vi "OAT Get Orbit Precession Direction.vi"(8 "error in (no error)":errorcluster, 9 "shaft rotating direction":u16, 10 "max data value":dbl format="%.2f", 11 "XY plot data in":cluster{dbl[], dbl[]}[](array[cluster]) {"?" format="%.2f"; "?" format="%.2f"}) -> (0 "error out":errorcluster, 3 "XY plot data out":cluster{dbl[], dbl[]}[](array[cluster]) {"?" format="%.2f"; "?" format="%.2f"})   [LabVIEW 2017]
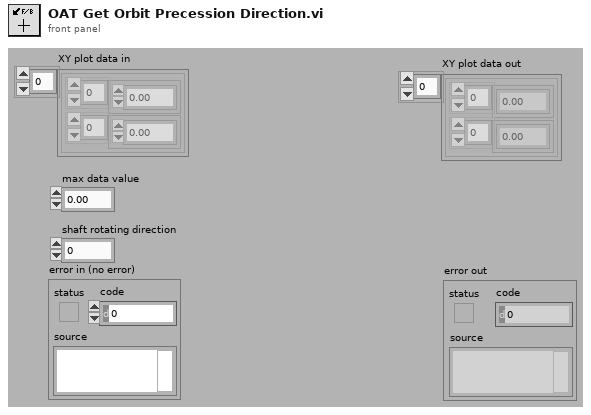
[diagram p1: front panel]
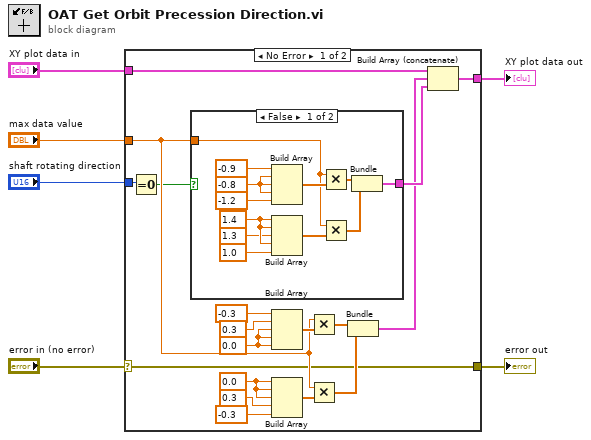
[diagram p0: block diagram]
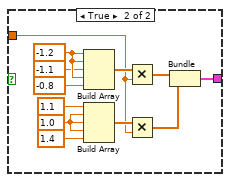
[diagram p2: hidden frame]
diagram:
  n1 = case shown="No Error" "error in (no error)" {
    selector: "error in (no error)" -> [w7 w50]
    tunnel: "XY plot data in" -> [w24 w49]
    tunnel: [w23 w49] -> w5
    tunnel: "max data value" -> [w12 _]
    tunnel: "shaft rotating direction" -> [w11 _]
    tunnel: [w7 w50] -> w1
    frame No Error {
      w16 = 0.0 ("x")
      w17 = 0.0 ("y")
      n2 = Equal To 0?(x=w11) -> (x = 0?=w10:bool)
      n3 = case shown="False" w10 {
        tunnel: [w36 w48] -> w9
        tunnel: w12 -> [w26 w39]
        frame False {
          w34 = -0.8 ("x")
          w32 = 1.4 ("x")
          n4 = Build Array(-0.9 ("x"), w34, w34, w34, -1.2 ("y")) -> (w29:dbl[])
          n5 = Build Array(w32, w32, 1.3 ("x"), w32, 1.0 ("x")) -> (w27:dbl[])
          n6 = Multiply(x=w26, y=w29) -> (x*y=w28:dbl[])
          n7 = Multiply(x=w26, y=w27) -> (x*y=w25:dbl[])
          n8 = Bundle(w28, w25) -> (w36:cluster{dbl[], dbl[]})  [unwired: 1 in]
        }
        frame True {
          w42 = 1.0 ("x")
          w47 = -1.2 ("x")
          n9 = Build Array(w47, w47, -1.1 ("x"), w47, -0.8 ("y")) -> (w41:dbl[])
          n10 = Build Array(1.1 ("x"), w42, w42, w42, 1.4 ("x")) -> (w40:dbl[])
          n11 = Multiply(x=w41, y=w39) -> (x*y=w38:dbl[])
          n12 = Multiply(x=w40, y=w39) -> (x*y=w37:dbl[])
          n13 = Bundle(w38, w37) -> (w48:cluster{dbl[], dbl[]})  [unwired: 1 in]
        }
      }
      n14 = Build Array(-0.3 ("x"), 0.3 ("x"), w17, w17, w17) -> (w21:dbl[])
      n15 = Build Array(w16, w16, w16, 0.3 ("x"), -0.3 ("x")) -> (w22:dbl[])
      n16 = Multiply(x=w12, y=w21) -> (x*y=w14:dbl[])
      n17 = Multiply(x=w12, y=w22) -> (x*y=w13:dbl[])
      n18 = Bundle(w14, w13) -> (w8:cluster{dbl[], dbl[]})  [unwired: 1 in]
      n19 = Build Array (concatenate)(w24, w8, w9) -> (w23:cluster{dbl[], dbl[]}[])
    }
    frame Error {
    }
  }
  "XY plot data out" <- w5
  "error out" <- w1
